vi "AlliGator Test Internal Data.vi"(6 "Test State":T1(ring), 8 "Error In":errorcluster, 11 "AlliGator Test Data":T2) -> (0 "Error Out":errorcluster, 3 "AlliGator Test Data":T2)   [LabVIEW 2021, in "AlliGator Test Suite.lvlib"]
doc: "Updates tested VI's error code."
uses:
  AlliGator Test Suite.lvlib
  AlliGator Test Data.ctl
panel:
  # "see the AlliGator License on the block diagram (Ctrl+E or Window:Show Block Diagram)"
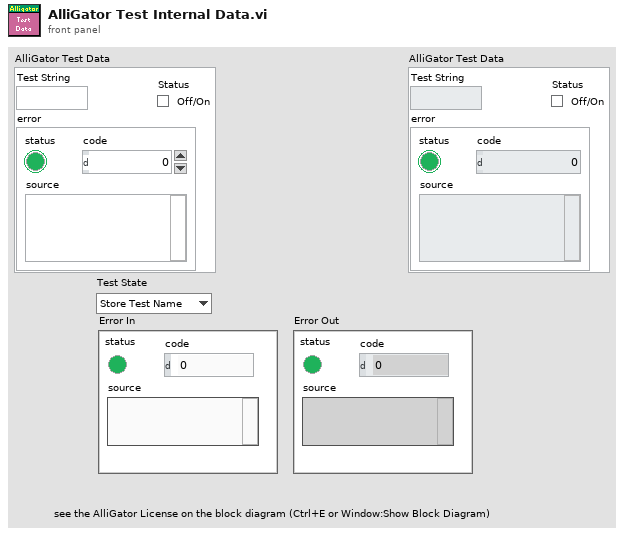
[diagram p1: front panel]
types:
  T1 = enum16{"Store Test Name", "Store Test Result", "Read Test Result"}
  T2 = typedef "AlliGator Test Suite.lvlib/AlliGator Test Data.ctl" = cluster{"Test String":string, "error":errorcluster, "Status":bool}
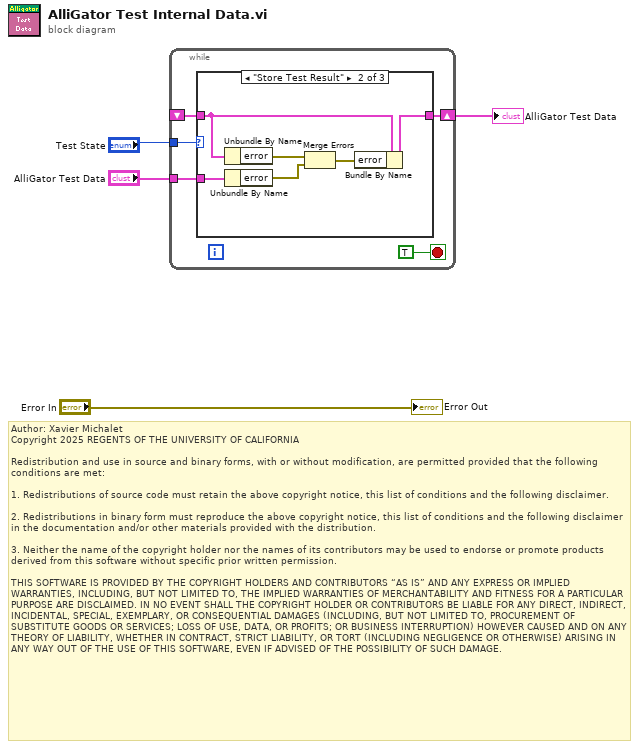
[diagram p0: block diagram]
diagram:
  # "Author: Xavier Michalet\nCopyright 2025 REGENTS OF THE UNIVERSITY OF CALIFORNIA\n\nRedistribution and use in source and binary forms, with or without modification, are permitted provided that the following conditions are met:\n\n1. Redistributions of source code must retain the above copyright notice, this list of conditions and the following disclaimer.\n\n2. Redistributions in binary form must reproduce the above copyright notice, this list of conditions and the following disclaimer in the documentation and/or other materials provided with the distribution.\n\n3. Neither the name of the copyright holder nor the names of its contributors may be used to endorse or promote products derived from this software without specific prior written permission.\n\nTHIS SOFTWARE IS PROVIDED BY THE COPYRIGHT HOLDERS AND CONTRIBUTORS “AS IS” AND ANY EXPRESS OR IMPLIED WARRANTIES, INCLUDING, BUT NOT LIMITED TO, THE IMPLIED WARRANTIES OF MERCHANTABILITY AND FITNESS FOR A PARTICULAR PURPOSE ARE DISCLAIMED. IN NO EVENT SHALL THE COPYRIGHT HOLDER OR CONTRIBUTORS BE LIABLE FOR ANY DIRECT, INDIRECT, INCIDENTAL, SPECIAL, EXEMPLARY, OR CONSEQUENTIAL DAMAGES (INCLUDING, BUT NOT LIMITED TO, PROCUREMENT OF SUBSTITUTE GOODS OR SERVICES; LOSS OF USE, DATA, OR PROFITS; OR BUSINESS INTERRUPTION) HOWEVER CAUSED AND ON ANY THEORY OF LIABILITY, WHETHER IN CONTRACT, STRICT LIABILITY, OR TORT (INCLUDING NEGLIGENCE OR OTHERWISE) ARISING IN ANY WAY OUT OF THE USE OF THIS SOFTWARE, EVEN IF ADVISED OF THE POSSIBILITY OF SUCH DAMAGE."
  n1 = while {
    tunnel: "Test State" -> [w8]
    shift-right: [w5] -> w1
    shift-left: _ -> [w6]
    tunnel: "AlliGator Test Data" -> [w7]
    stop <- TRUE stop-if-true
    n2 = case shown="\"Store Test Result\"" w8 {
      tunnel: w7 -> [w10 w16 _]
      tunnel: w6 -> [_ w12 w17]
      tunnel: [w10 w15 w17] -> w5
      frame "Store Test Name", Default {
      }
      frame "Store Test Result" {
        n3 = Unbundle By Name(w12) -> ("error"=w14:errorcluster)
        n4 = Unbundle By Name(w16) -> ("error"=w13:errorcluster)
        n5 = Merge Errors(w14, w13) -> (w11:errorcluster)
        n6 = Bundle By Name(cluster=w12, "error"=w11) -> (w15:T2)
      }
      frame "Read Test Result" {
      }
    }
  }
  "AlliGator Test Data" <- w1
  "Error Out" <- "Error In"
